vi "keithley-2400_sweep.vi"(4 "Timeout (ms)":i32=10000000, 5 "Sweep Direction":u16(ring) items=["Low to high", "High to low"], 6 "Number of Points":u32=5, 7 "Maximum Amplitude":dbl=2.0, 8 "Minimum Amplitude":dbl=1.0, 9 "VISA resource name out 2":refnum<visa-resource-name>) -> (0 "Measurement Complete":bool, 2 "Data Array":dbl[][](array[numeric]), 3 "VISA resource name out":refnum<visa-resource-name>)   [LabVIEW 2016]
doc: "Configures a sweep and takes voltage and current readings at each point."
uses:
  <instrlib>/Keithley 24XX/Public/Data/Read (Multiple Points).vi
  <instrlib>/Keithley 24XX/Keithley 24XX.lvlib
panel:
  in  "Source Mode  (0: Voltage)":u16(ring) items=["Voltage", "Current"]
  # "(c) 2006 National Instruments.  ALL RIGHTS RESERVED."
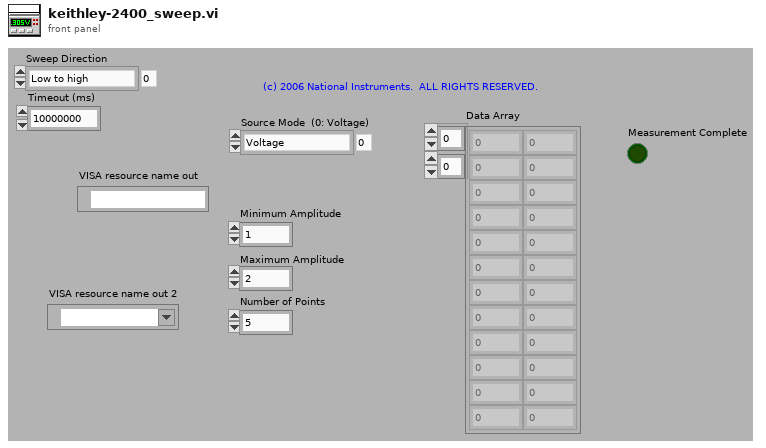
[diagram p1: front panel]
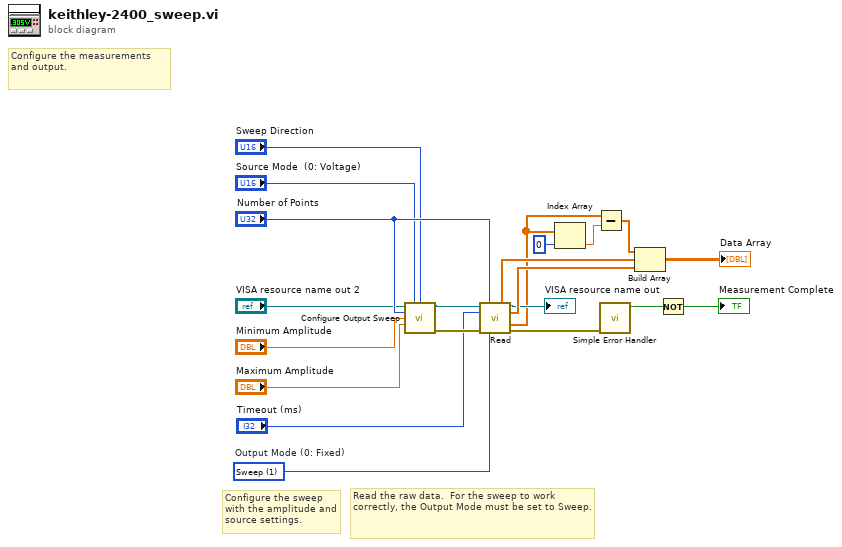
[diagram p0: block diagram]
diagram:
  w16 = u16 1 items=["Fixed", "Sweep", "List"]  # Output Mode (0: Fixed)
  # "Read the raw data.  For the sweep to work correctly, the Output Mode must be set to Sweep."
  # "Configure the sweep with the amplitude and source settings."
  # "Configure the measurements and output."
  n1 = call <instrlib>:"Configure Output Sweep.vi"("VISA resource name"="VISA resource name out 2", "Source Mode  (0: Voltage)"="Source Mode  (0: Voltage)", "Sweep Direction  (0: Ascending)"="Sweep Direction", "Number of Points (5)"="Number of Points", "Minimum Amplitude (1)"="Minimum Amplitude", "Maximum Amplitude (2)"="Maximum Amplitude") -> ("VISA resource name out"=w7:refnum<visa-resource-name>, "error out"=w6:errorcluster)  [unwired: 8 in]
  n2 = call-poly <instrlib>:"Read.vi"("VISA resource name"=w7, "Sample Count (1)"="Number of Points", "Timeout (10000 ms)"="Timeout (ms)", "error in (no error)"=w6, "Output Mode (0: Fixed)"=w16) -> ("Voltage"=w19:sgl[], "VISA resource name out"=→"VISA resource name out":refnum<visa-resource-name>, "Current"=w18:sgl[], "Timestamp"=w3:sgl[], "error out"=w14:errorcluster)  [unwired: 4 in, 2 out]
  n3 = Index Array(array=w3, index=0) -> (element=w2:sgl)
  n4 = Subtract(x=w3, y=w2) -> (x-y=w1:sgl[])
  n5 = call <vilib>:"Simple Error Handler.vi"("error in (no error)"=w14) -> ("error?"=w12:bool)  [unwired: 4 in, 4 out]
  n6 = Build Array(w1, w19, w18) -> (→"Data Array":sgl[][])
  n7 = Not(x=w12) -> (.not. x?=→"Measurement Complete":bool)
